vi "PM100D_GetRngIndex.vi"(5 "error in (no error)":errorcluster, 11 "VISA in":refnum<visa-resource-name>) -> (0 "error out":errorcluster, 1 "SensType":i32 min=0 max=3, 2 "Rng_Array":string[](array[string]), 3 "dup VISA session":refnum<visa-resource-name>, 4 "IndexOut":i32, 9 "AutoOut":bool)   [LabVIEW 2011]
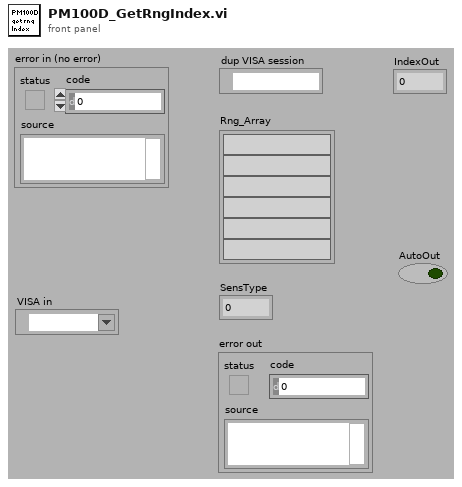
[diagram p1: front panel]
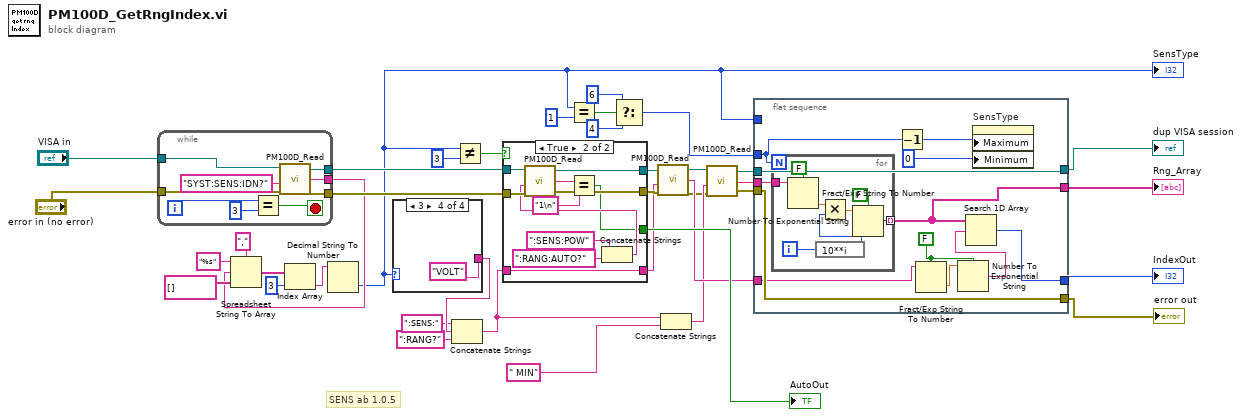
[diagram p0: block diagram]
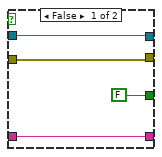
[diagram p2: hidden frame]
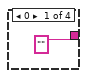
[diagram p3: hidden frame]
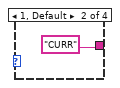
[diagram p4: hidden frame]
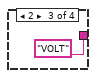
[diagram p5: hidden frame]
diagram:
  # "SENS ab 1.0.5"
  n1 = while {
    tunnel: [w48] -> w35
    tunnel: [w47] -> w33
    tunnel: [w45] -> w27
    tunnel: "error in (no error)" -> [w44]
    tunnel: "VISA in" -> [w43]
    i -> [w41]
    stop <- w42 stop-if-true
    n2 = Equal?(x=w41, y=3) -> (x = y?=w42:bool)
    n3 = call "PM100D_Read.vi"("error in (no error)"=w44, "Command"="SYST:SENS:IDN?", "VISA in"=w43) -> ("error out"=w48:errorcluster, "ReadValue"=w45:string, "VISA out"=w47:refnum<visa-resource-name>)  [unwired: 1 in]
  }
  n4 = Spreadsheet String To Array(delimiter (Tab)=",", format string="%s", spreadsheet string=w27, array type (2D Dbl)=string[] [] ("Rng_Array")) -> (array=w29:string[])
  n5 = Index Array(array=w29, index=3) -> (element=w32:string)
  n6 = Decimal String To Number(string=w32) -> (number=w5:i32)  [unwired: 2 in, 1 out]
  "SensType" <- w5
  n7 = case shown="3" w5 {
    tunnel: ["" "CURR" "VOLT" "VOLT"] -> w21
    frame 0 {
    }
    frame 1, Default {
    }
    frame 2 {
    }
    frame 3 {
    }
  }
  n8 = Concatenate Strings(":SENS:" ("string"), w21, ":RANG?" ("string")) -> (w2:string)
  n9 = Not Equal?(x=w5, y=3) -> (x != y?=w38:bool)
  n10 = case shown="True" w38 {
    tunnel: w33 -> [w56 w67]
    tunnel: [w56 w66] -> w34
    tunnel: w35 -> [w55 w65]
    tunnel: [w55 w64] -> w36
    tunnel: [FALSE w58] -> w39
    tunnel: w2 -> [w53 w57]
    tunnel: [w53 w57] -> w1
    frame False {
    }
    frame True {
      n11 = Concatenate Strings(":SENS:POW" ("string"), ":RANG:AUTO?" ("string")) -> (w63:string)
      n12 = call "PM100D_Read.vi"("error in (no error)"=w65, "Command"=w63, "VISA in"=w67) -> ("error out"=w64:errorcluster, "ReadValue"=w60:string, "VISA out"=w66:refnum<visa-resource-name>)  [unwired: 1 in]
      n13 = Equal?(x=w60, y="1\n") -> (x = y?=w58:bool)
    }
  }
  "AutoOut" <- w39
  n14 = Equal?(x=w5, y=1) -> (x = y?=w23:bool)
  n15 = Select(t=6, s=w23, f=4) -> (s? t:f=w12:i32)
  n16 = call "PM100D_Read.vi"("error in (no error)"=w36, "Command"=w1, "VISA in"=w34) -> ("error out"=w8:errorcluster, "ReadValue"=w18:string, "VISA out"=w7:refnum<visa-resource-name>)  [unwired: 1 in]
  n17 = Concatenate Strings(w2, " MIN" ("string")) -> (w10:string)
  n18 = call "PM100D_Read.vi"("error in (no error)"=w8, "Command"=w10, "VISA in"=w7) -> ("error out"=w16:errorcluster, "ReadValue"=w17:string, "VISA out"=w15:refnum<visa-resource-name>)  [unwired: 1 in]
  n19 = flat-sequence {
    tunnel: w12 -> [w71]
    tunnel: w15 -> [w79]
    tunnel: [w79] -> w19
    tunnel: [w78] -> w20
    tunnel: w16 -> [w78]
    tunnel: w17 -> [w77]
    tunnel: w18 -> [w76]
    tunnel: [w72] -> w6
    tunnel: [w70] -> w4
    tunnel: w5 -> [_]
    frame #0 {
      w74 = FALSE ("use system decimal point (T)")
      n20 = for {
        N: w71 -> [_]
        tunnel: w77 -> [w86]
        tunnel: [w80] -> w72 mode=indexing
        i -> [w87]
        n21 = Fract/Exp String To Number(use system decimal point (T)=FALSE, string=w86) -> (number=w85:dbl)  [unwired: 2 in, 1 out]
        n22 = expression code="10**i"(w87) -> (w84:i32)
        n23 = Multiply(x=w85, y=w84) -> (x*y=w82:dbl)
        n24 = Number To Exponential String(number=w82, 1:FALSE ("use system decimal point (T)")) -> (E-format string=w80:string)  [unwired: 2 in]
      }
      n25 = Decrement(x=w71) -> (x-1=w69:i32)
      n26 = Fract/Exp String To Number(use system decimal point (T)=w74, string=w76) -> (number=w75:dbl)  [unwired: 2 in, 1 out]
      n27 = Number To Exponential String(number=w75, 1:w74) -> (E-format string=w73:string)  [unwired: 2 in]
      n28 = Search 1D Array(1D array=w72, element=w73) -> (index of element=w70:i32)  [unwired: 1 in]
      n29 = property on="SensType" class="DigNum (strict)"("Maximum"=w69, "Minimum"=0) -> ()  [unwired: 2 in, 2 out]
    }
  }
  "Rng_Array" <- w6
  "error out" <- w20
  "dup VISA session" <- w19
  "IndexOut" <- w4
